vi "AUX device cluster to String.vi"(11 "Auxiliary Device":T1 {"Signals"."% Open" min=0.0 max=100.0 step=0.1 format="%#.1f"; "Speed" max=7 step=1; "Gear" max=7 step=1; "Temp V Err" min=0.0 max=20.0 step=0.1; "Temp Err" min=0.0 max=20.0 step=0.1; "Scaling Factor" min=0.0 max=99.0 step=0.1; "Min Flow" min=0.0 max=20.0 step=0.1}) -> (3 "Data to send":string=":GMIN:1.1:GFSF:1.5:TES:2.0:TVES:2.5:GEAR:3:SPD:1:SIG:OPEN:50.0:SIG")   [LabVIEW 2013, in "Mercury iXX.lvlib" / "Auxiliary.lvlib"]
uses:
  <instrlib>/Mercury iXX/Public/Libraries/Auxiliary.lvlib
  <instrlib>/Mercury iXX/Public/Libraries/Auxiliary/Controls/AUX Device (Set).ctl
  <instrlib>/Mercury iXX/Public/Libraries/Auxiliary/Controls/AUX Signals (Set).ctl
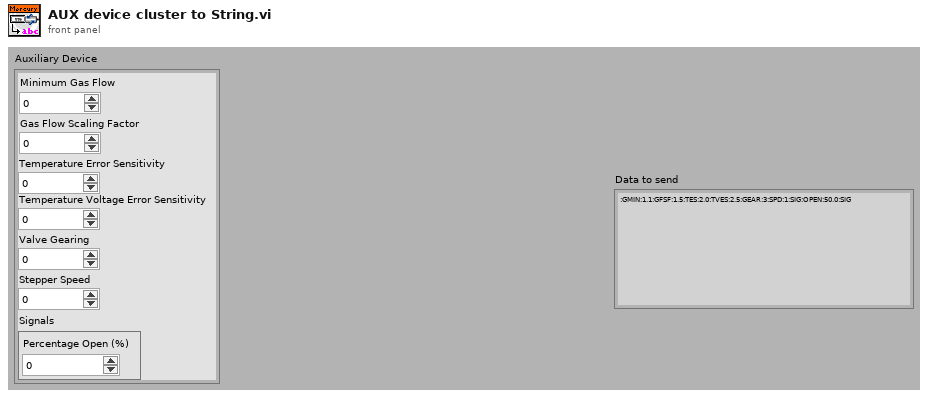
[diagram p1: front panel]
types:
  T1 = typedef "Mercury iXX.lvlib/Auxiliary.lvlib/AUX Device (Set).ctl" = cluster{"Min Flow":dbl, "Scaling Factor":dbl, "Temp Err":dbl, "Temp V Err":dbl, "Gear":u32, "Speed":u32, "Signals":T2}
  T2 = typedef "Mercury iXX.lvlib/Auxiliary.lvlib/AUX Signals (Set).ctl" = cluster{"% Open":dbl}
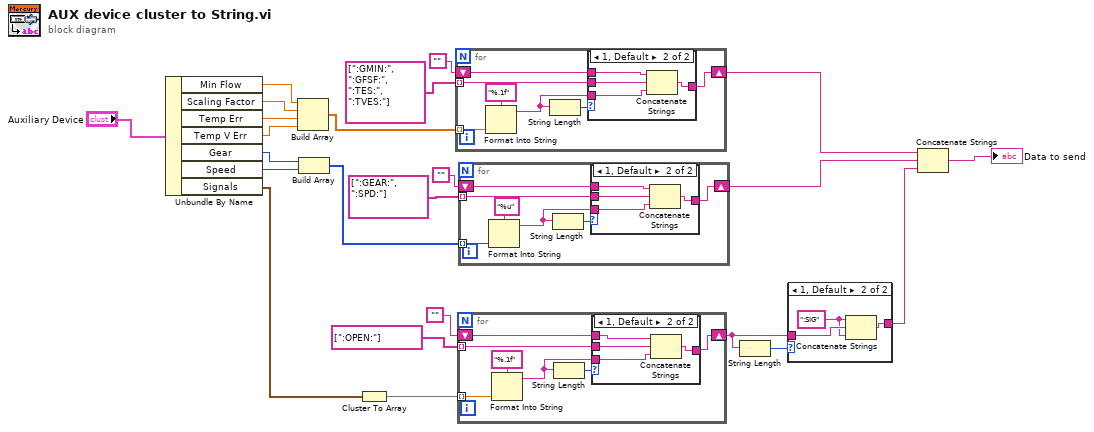
[diagram p0: block diagram]
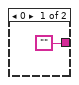
[diagram p3: hidden frame]
diagram:
  n1 = Unbundle By Name("Auxiliary Device") -> ("Min Flow"=w13:dbl, "Scaling Factor"=w14:dbl, "Temp Err"=w22:dbl, "Temp V Err"=w6:dbl, "Gear"=w5:u32, "Speed"=w4:u32, "Signals"=w9:T2)
  n2 = Build Array(w13, w14, w22, w6) -> (w12:dbl[])
  n3 = Build Array(w5, w4) -> (w3:u32[])
  n4 = Cluster To Array(cluster=w9) -> (array=w18:dbl[])
  n5 = for {
    tunnel: w12 -> [w26] mode=indexing
    tunnel: string[] [":GMIN:", ":GFSF:", ":TES:", ":TVES:"] ("Excitation") -> [w29] mode=indexing
    shift-right: [w28] -> w15
    shift-left: "" -> [w27]
    n6 = Format Into String(format string="%.1f", w26) -> (resulting string=w25:string)  [unwired: 2 in, 1 out]
    n7 = String Length(string=w25) -> (length=w30:i32)
    n8 = case shown="1, Default" w30 {
      tunnel: w25 -> [_ w34]
      tunnel: [w31 w35] -> w28
      tunnel: w29 -> [_ w33]
      tunnel: w27 -> [w31 w32]
      frame 0 {
      }
      frame 1, Default {
        n9 = Concatenate Strings(w32, w33, w34) -> (w35:string)
      }
    }
  }
  n10 = for {
    tunnel: w18 -> [w36] mode=indexing
    tunnel: string[] [":OPEN:"] ("Excitation") -> [w41] mode=indexing
    shift-right: [w39] -> w11
    shift-left: "" -> [w40]
    n11 = Format Into String(format string="%.1f", w36) -> (resulting string=w37:string)  [unwired: 2 in, 1 out]
    n12 = String Length(string=w37) -> (length=w42:i32)
    n13 = case shown="1, Default" w42 {
      tunnel: w37 -> [_ w46]
      tunnel: [w43 w47] -> w39
      tunnel: w41 -> [_ w45]
      tunnel: w40 -> [w43 w44]
      frame 0 {
      }
      frame 1, Default {
        n14 = Concatenate Strings(w44, w45, w46) -> (w47:string)
      }
    }
  }
  n15 = for {
    tunnel: w3 -> [w50] mode=indexing
    tunnel: string[] [":GEAR:", ":SPD:"] ("Excitation") -> [w53] mode=indexing
    shift-right: [w52] -> w1
    shift-left: "" -> [w51]
    n16 = Format Into String(format string="%u", w50) -> (resulting string=w49:string)  [unwired: 2 in, 1 out]
    n17 = String Length(string=w49) -> (length=w54:i32)
    n18 = case shown="1, Default" w54 {
      tunnel: w49 -> [_ w58]
      tunnel: [w55 w59] -> w52
      tunnel: w53 -> [_ w57]
      tunnel: w51 -> [w55 w56]
      frame 0 {
      }
      frame 1, Default {
        n19 = Concatenate Strings(w56, w57, w58) -> (w59:string)
      }
    }
  }
  n20 = String Length(string=w11) -> (length=w10:i32)
  n21 = case shown="1, Default" w10 {
    tunnel: ["" w63] -> w2
    tunnel: w11 -> [_ w62]
    frame 0 {
    }
    frame 1, Default {
      w61 = ":SIG" ("string")
      n22 = Concatenate Strings(w61, w62, w61) -> (w63:string)
    }
  }
  n23 = Concatenate Strings(w15, w1, w2) -> (→"Data to send":string)
